vi "Initialize DAQ.vi"(8 "error in (no error)":errorcluster, 11 "Acq and Logging Props":T1) -> (0 "error out":errorcluster, 3 "DAQmx Task Name":refnum<k21>)   [LabVIEW 2013]
uses:
  <vilib>/DAQmx/create/channels.llb/DAQmx Create Channel (AI-Voltage-Basic).vi
  <vilib>/DAQmx/configure/timing.llb/DAQmx Timing (Sample Clock).vi
  <resource>/objmgr/daqmx.rc
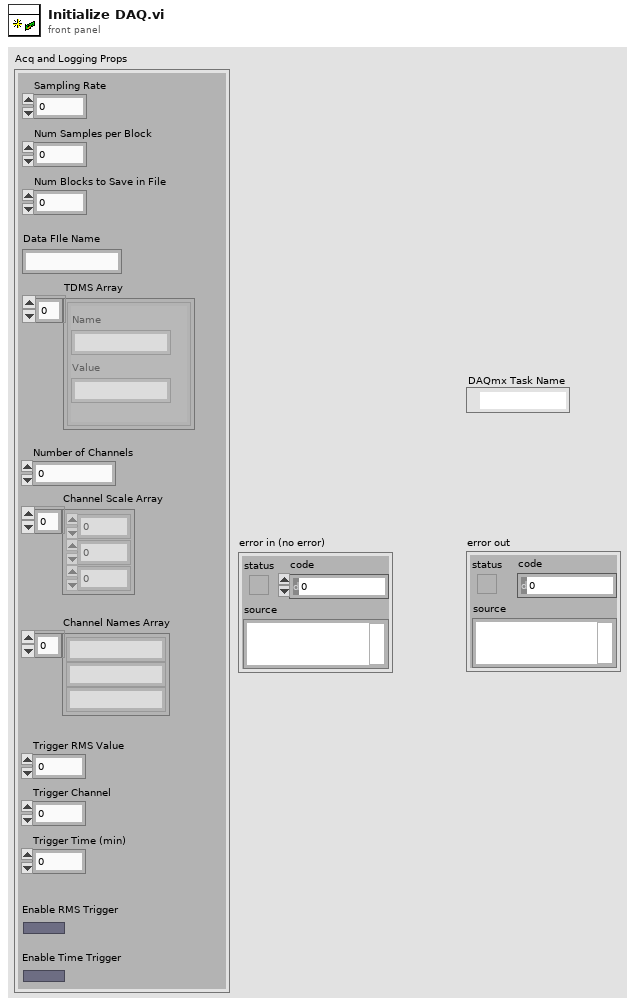
[diagram p1: front panel]
types:
  T1 = cluster{"Sampling Rate":dbl, "Num Samples per Block":i32, "Num Blocks to Save in File":i32, "Data FIle Name":string, "TDMS Array":cluster{"Name":string, "Value":string}[], "Number of Channels":i32, "Channel Scale Array":dbl[], "Channel Names Array":string[], "Trigger RMS Value":dbl, "Trigger Channel":i32, "Trigger Time (min)":i32, "Enable RMS Trigger":bool, "Enable Time Trigger":bool}
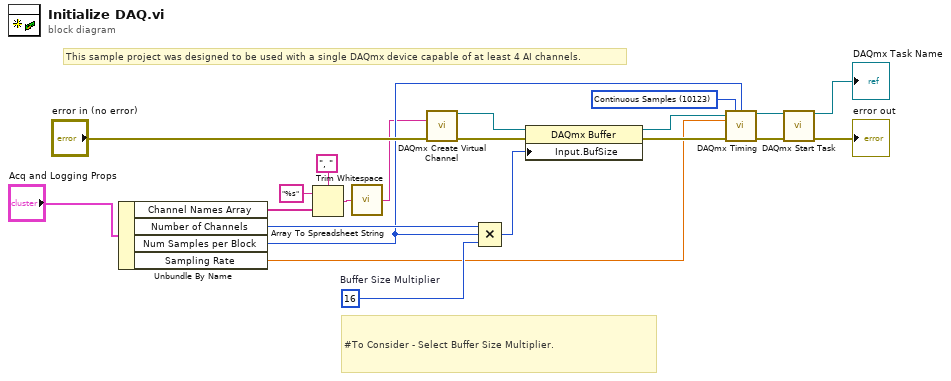
[diagram p0: block diagram]
diagram:
  w8 = 10123 items=["Finite Samples"=10178, "Continuous Samples"=10123, "Hardware Timed Single Point"=12522] ("sample mode")
  w14 = 16  # Buffer Size Multiplier
  # "This sample project was designed to be used with a single DAQmx device capable of at least 4 AI channels."
  # "#To Consider - Select Buffer Size Multiplier."
  n1 = Unbundle By Name("Acq and Logging Props") -> ("Channel Names Array"=w20:string[], "Number of Channels"=w15:i32, "Num Samples per Block"=w7:i32, "Sampling Rate"=w6:dbl)
  n2 = Array To Spreadsheet String(delimiter (Tab)=", ", array=w20, 3:"%s" ("format string")) -> (spreadsheet string=w3:string)
  n3 = call <vilib>:"Trim Whitespace.vi"("string"=w3) -> ("trimmed string"=w2:string)  [unwired: 1 in]
  n4 = call-poly <vilib>:"DAQmx Create Virtual Channel.vi"("physical channels"=w2, "error in"="error in (no error)") -> ("task out"=w16:refnum<k21>, "error out"=w17:errorcluster)  [unwired: 12 in]
  n5 = Compound Arithmetic op=MULTIPLY(w15, w7, w14) -> (w13:i32)
  n6 = property class="DAQmx Buffer"(reference=w16, error in=w17, "Input.BufSize"=w13) -> (reference out=w9:refnum<k21>, error out=w10:errorcluster)
  n7 = call-poly <vilib>:"DAQmx Timing.vi"("task/channels in"=w9, "sample mode"=w8, "samples per channel"=w7, "rate"=w6, "error in"=w10) -> ("task out"=w11:refnum<k21>, "error out"=w12:errorcluster)  [unwired: 9 in]
  n8 = call <vilib>:"DAQmx Start Task.vi"("task/channels in"=w11, "error in"=w12) -> ("task out"=→"DAQmx Task Name":refnum<k21>, "error out"=→"error out":errorcluster)  [unwired: 12 in]
